vi "Query Registered Instruction.vi"(8 "error in (no error)":errorcluster, 10 "Motor ID (0)":u8, 11 "VISA resource name":refnum<visa-resource-name>) -> (0 "error out":errorcluster, 2 "Registered Instruction":bool, 3 "VISA resource name out":refnum<visa-resource-name>)   [LabVIEW 2016, in "Dynamixel Motor.lvlib"]
doc: "Queries the motor to see if it has an instruction registered. This would indicate that a registered write command was used. The write to the motor's register will not be carried out until an Action command is issued."
uses:
  Dynamixel Motor.lvlib
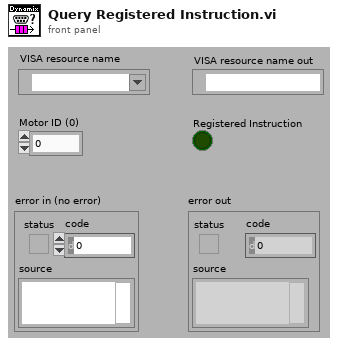
[diagram p1: front panel]
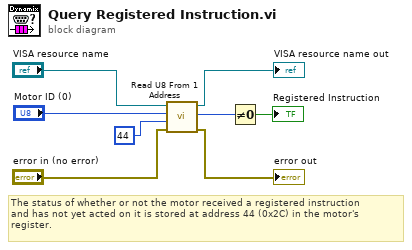
[diagram p0: block diagram]
diagram:
  # "The status of whether or not the motor received a registered instruction\nand has not yet acted on it is stored at address 44 (0x2C) in the motor's\nregister."
  n1 = call "Read U8 From 1 Address.vi"("Error in (no error)"="error in (no error)", "Address number (0)"=u8 44 ("Address # DEC"), "Motor ID (0)"="Motor ID (0)", "VISA resource name"="VISA resource name") -> ("error out"=→"error out":errorcluster, "Data"=w4:u8, "VISA resource name out"=→"VISA resource name out":refnum<visa-resource-name>)  [unwired: 5 in]
  n2 = Not Equal To 0?(x=w4) -> (x != 0?=→"Registered Instruction":bool)
